vi "220407_Basic2.vi"() -> ()   [LabVIEW 2021]
uses:
  <vilib>/numeric/Random Number (Range) U64.vi
  f5532365-0c95-4832-9939-820343218a1b.vi
panel:
  out "Sorted Random  2":u64[](array[numeric])
  out "Joker":string
  out "Joker":u64[](array[numeric])
  out "Sorted Random":dbl[](array[numeric])
  out "Random over 15":u64[](array[numeric])
  out "Random":u64[](array[numeric])
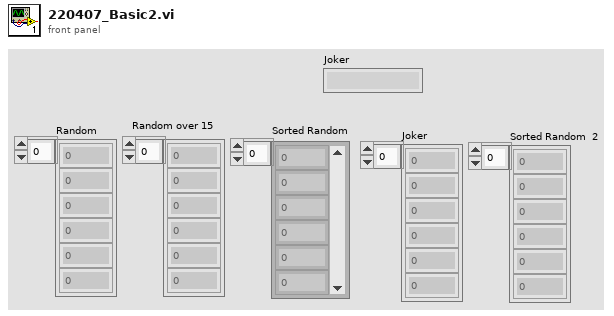
[diagram p1: front panel]
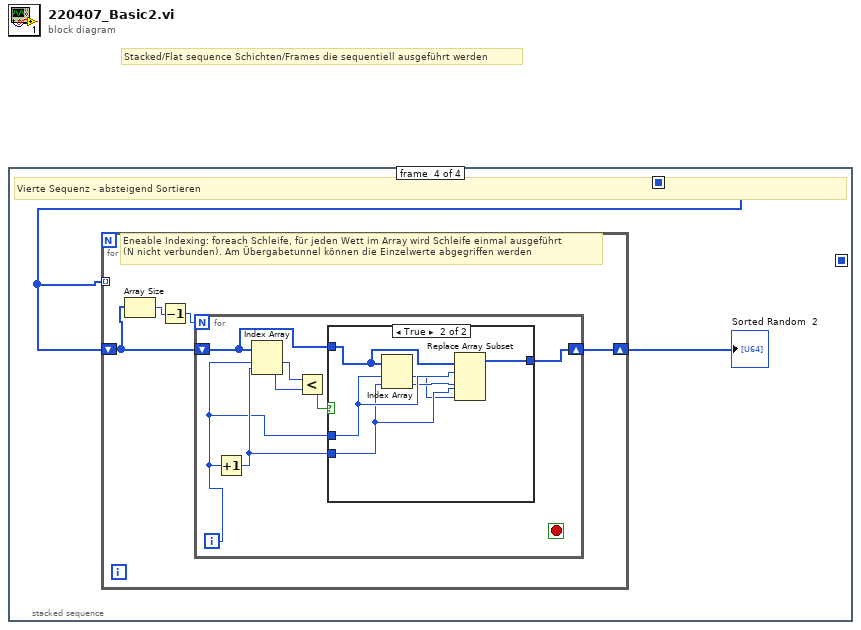
[diagram p0: block diagram]
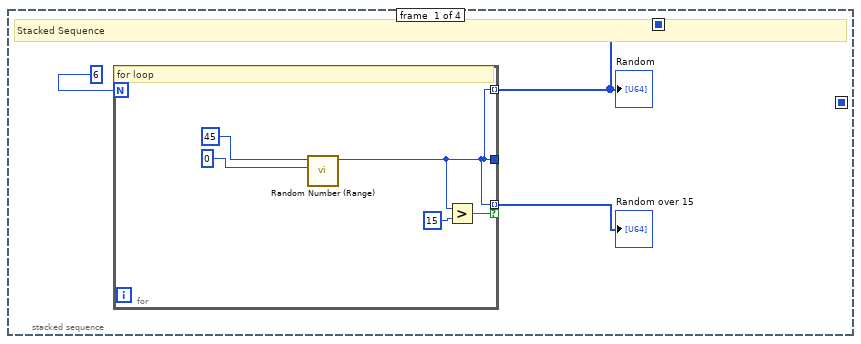
[diagram p2: hidden frame]
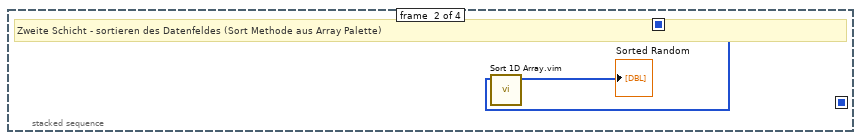
[diagram p3: hidden frame]
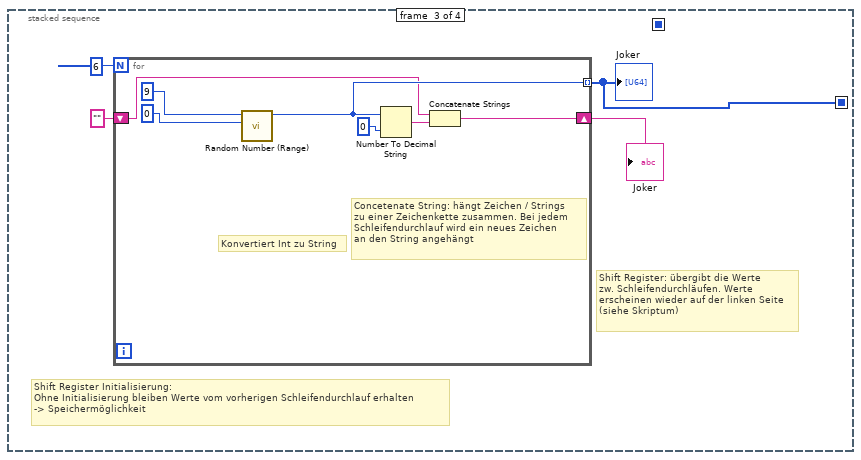
[diagram p4: hidden frame]
diagram:
  # "Stacked/Flat sequence Schichten/Frames die sequentiell ausgeführt werden"
  n1 = stacked-sequence {
    seq-local: [w1 _ _ _] -> [_ w10 _ w22]
    seq-local: [_ _ w11 _] -> [_ _ _ _]
    frame #0 {
      # "Stacked Sequence"
      n2 = for {
        N: 6 -> [_]
        tunnel: [w6] -> w1 mode=indexing
        tunnel: [w6] -> _
        tunnel: [w6] -> w2 mode=indexing if=w5
        # "for loop"
        n3 = call-poly <vilib>:"Random Number (Range).vi"("lower bound (0)"=u64 0, "upper bound (100)"=u64 45) -> ("number"=w6:u64)  [unwired: 9 in]
        n4 = Greater?(x=w6, y=u64 15) -> (0:w5:bool)
      }
      "Random" <- w1
      "Random over 15" <- w2
    }
    frame #1 {
      # "Zweite Schicht - sortieren des Datenfeldes (Sort Methode aus Array Palette)"
      n5 = call "Sort 1D Array.vim"("unsorted array"=w10) -> ("sorted array"=→"Sorted Random":u64[])  [unwired: 10 in]
    }
    frame #2 {
      # "Shift Register Initialisierung:\nOhne Initialisierung bleiben Werte vom vorherigen Schleifendurchlauf erhalten\n-> Speichermöglichkeit"
      # "Shift Register: übergibt die Werte \nzw. Schleifendurchläufen. Werte\nerscheinen wieder auf der linken Seite\n(siehe Skriptum)"
      n6 = for {
        N: 6 -> [_]
        tunnel: [w18] -> w11 mode=indexing
        shift-right: [w15] -> w13
        shift-left: "" -> [w17]
        # "Konvertiert Int zu String"
        # "Concetenate String: hängt Zeichen / Strings\nzu einer Zeichenkette zusammen. Bei jedem\nSchleifendurchlauf wird ein neues Zeichen\nan den String angehängt"
        n7 = call-poly <vilib>:"Random Number (Range).vi"("lower bound (0)"=u64 0, "upper bound (100)"=u64 9) -> ("number"=w18:u64)  [unwired: 9 in]
        n8 = Number To Decimal String(number=w18, width (-)=i16 0) -> (decimal integer string=w16:string)
        n9 = Concatenate Strings(w17, w16) -> (w15:string)
      }
      "Joker" <- w11
      "Joker" <- w13
    }
    frame #3 {
      # "Vierte Sequenz - absteigend Sortieren"
      n10 = for {
        shift-right: [w27] -> w23
        shift-left: w22 -> [w24]
        tunnel: w22 -> [_] mode=indexing
        # "Eneable Indexing: foreach Schleife, für jeden Wett im Array wird Schleife einmal ausgeführt\n(N nicht verbunden). Am Übergabetunnel können die Einzelwerte abgegriffen werden"
        n11 = Array Size(array=w24) -> (size(s)=w26:i32)
        n12 = Decrement(x=w26) -> (x-1=w25:i32)
        n13 = for {
          N: w25 -> [_]
          shift-right: [w33] -> w27
          shift-left: w24 -> [w34]
          i -> [w31]
          stop <- _ stop-if-true
          n14 = Increment(x=w31) -> (x+1=w32:i32)
          n15 = Index Array(array=w34, index #1=w31, index #2=w32) -> (element #1=w30:u64, element #2=w29:u64)
          n16 = Less?(x=w30, y=w29) -> (x < y?=w28:bool)
          n17 = case shown="True" w28 {
            tunnel: w34 -> [w35 w41]
            tunnel: w31 -> [_ w40]
            tunnel: w32 -> [_ w39]
            tunnel: [w35 w36] -> w33
            frame False {
            }
            frame True {
              n18 = Index Array(array=w41, index #1=w40, index #2=w39) -> (element #1=w37:u64, element #2=w38:u64)
              n19 = Replace Array Subset(array=w41, new element #1=w38, index #1=w40, new element #2=w37, index #2=w39) -> (w36:u64[])
            }
          }
        }
      }
      "Sorted Random  2" <- w23
    }
  }
